vi "Change Setting.vi"(8 "error in (no error)":errorcluster, 10 "Change setting mode":T1=enum."Next", 11 "Device in":refnum<class "Device.lvclass">) -> (0 "error out":errorcluster, 1 "Changes":cluster{"Name":string, "Value":string}[](array[cluster]), 2 "Last setting":bool, 3 "Device out":refnum<class "Device.lvclass">)   [LabVIEW 2020, in "Device.lvclass"]
uses:
  Device.lvclass
  Controls/Change setting mode enum.ctl
  PIC-device/PIC-Device.lvclass
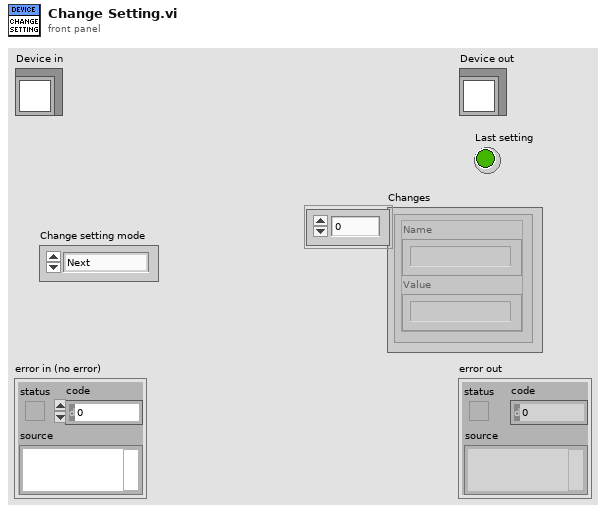
[diagram p1: front panel]
types:
  T1 = typedef "PIC-Device.lvclass/Change setting mode enum.ctl" = enum16{"Init", "Next", "Reset"}
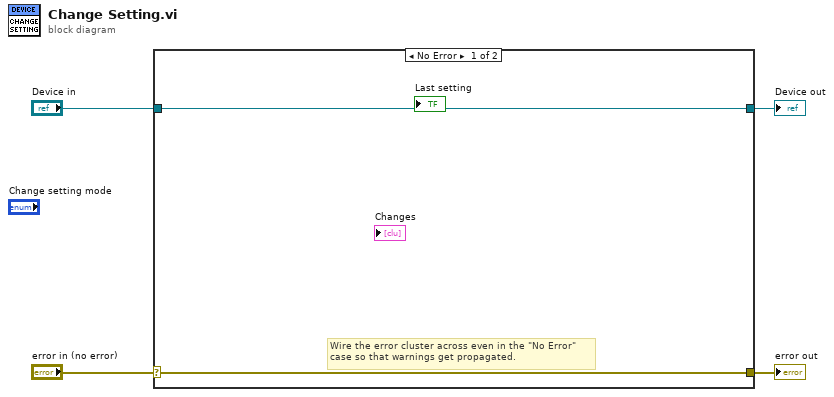
[diagram p0: block diagram]
diagram:
  n1 = case shown="No Error" "error in (no error)" {
    selector: "error in (no error)" -> [w5 w8]
    tunnel: [w5 w8] -> w3
    tunnel: [w6 w7] -> w1
    tunnel: "Device in" -> [w6 w7]
    frame No Error {
      # "Wire the error cluster across even in the \"No Error\"\ncase so that warnings get propagated."
    }
    frame Error {
    }
  }
  "error out" <- w3
  "Device out" <- w1
